vi "Configure IQ Recorder Measurement Write Results To IQ File.vi"(8 "error in (no error)":errorcluster, 9 "Write To IQ File (Off)":i32(ring) items=["Off", "On", "Only"], 10 "Instance (1)":i32=1, 11 "VISA resource name":refnum<visa-resource-name>) -> (0 "error out":errorcluster, 3 "VISA resource name out":refnum<visa-resource-name>)   [LabVIEW 2020, in "Rohde&Schwarz CMXP GPRF.lvlib"]
doc: "This VI selects whether the results are written to an I/Q file, to the memory or both.\n\nAttribute:\nRSCMXPGPRF_ATTR_IQ_RECORDER_MEASUREMENT_WRITE_RESULT_TO_IQ_FILE\n\nRemote-control command:\nCONFigure:GPRF:MEAS<i>:IQRecorder:WTFile"
uses:
  <instrlib>/Rohde&Schwarz CMXP GPRF/Rohde&Schwarz CMXP GPRF.lvlib
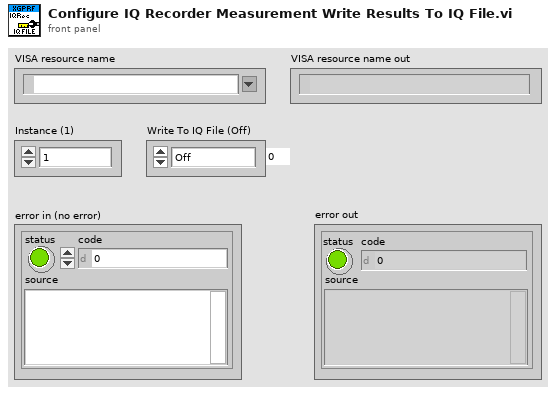
[diagram p1: front panel]
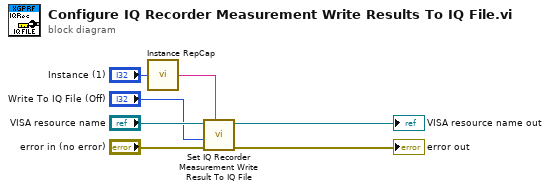
[diagram p0: block diagram]
diagram:
  n1 = call <instrlib>:"Instance RepCap.vi"("Instance in"="Instance (1)") -> ("Instance out"=w2:string)
  n2 = call "Set IQ Recorder Measurement Write Result To IQ File"("Repeated Capabilities"=w2, "error in (no error)"="error in (no error)", "IQ Recorder Measurement Write Result To IQ File (0 - Off)"="Write To IQ File (Off)", "instrument handle"="VISA resource name") -> ("error out"=→"error out":errorcluster, "instrument handle out"=→"VISA resource name out":refnum<visa-resource-name>)  [unwired: 6 in]
